vi "PC_NS_Signal disconnect_communication.vi"(8 "error in (no error)":errorcluster, 11 "PC_NS_Signal in":refnum<class "PC_NS_Signal.lvclass">) -> (0 "error out":errorcluster, 3 "PC_NS_Signal out":refnum<class "PC_NS_Signal.lvclass">)   [LabVIEW 2018, in "PC_NS_Signal.lvclass"]
uses:
  PC_NS_Signal.lvclass
  PC_NS_Signal.lvclass/PC_NS_Signal.ctl
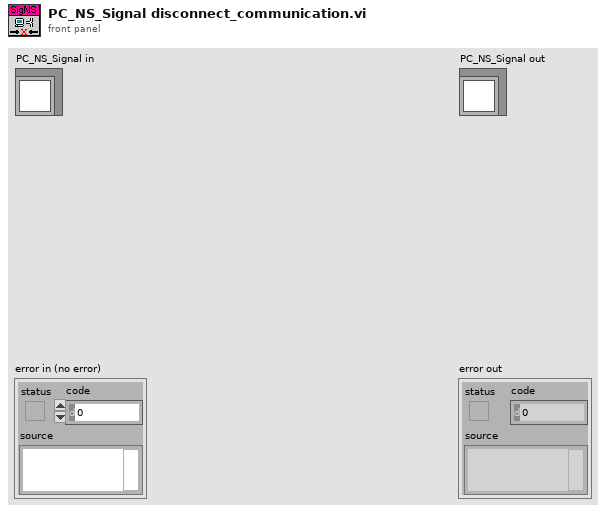
[diagram p1: front panel]
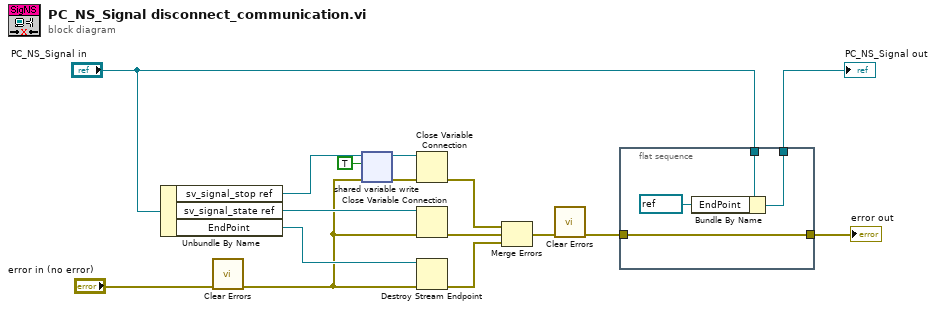
[diagram p0: block diagram]
diagram:
  n1 = Unbundle By Name("PC_NS_Signal in") -> ("sv_signal_stop ref"=w6:refnum<k21>, "sv_signal_state ref"=w16:refnum<k21>, "EndPoint"=w2:refnum<k21>)
  n2 = call <vilib>:"Clear Errors.vi"("error in (no error)"="error in (no error)") -> ("error out"=w1:errorcluster)  [unwired: 5 in, 1 out]
  n3 = shared-variable-write(w6, w1, TRUE ("data in")) -> (w4:refnum<k21>, w3:errorcluster)
  n4 = Close Variable Connection(8:w3, 11:w4) -> (0:w15:errorcluster)
  n5 = Close Variable Connection(8:w1, 11:w16) -> (0:w14:errorcluster)
  n6 = Destroy Stream Endpoint(8:w1, 11:w2) -> (0:w13:errorcluster)
  n7 = Merge Errors(w15, w14, w13) -> (w12:errorcluster)
  n8 = call <vilib>:"Clear Errors.vi"("error in (no error)"=w12) -> ("error out"=w8:errorcluster)  [unwired: 5 in, 1 out]
  n9 = flat-sequence {
    tunnel: "PC_NS_Signal in" -> [w20]
    tunnel: [w19] -> w9
    tunnel: w8 -> [w17]
    tunnel: [w17] -> w7
    frame #0 {
      n10 = Bundle By Name(cluster=w20, "EndPoint"=refnum<k21> refnum) -> (w19:refnum<class "PC_NS_Signal.lvclass">)
    }
  }
  "error out" <- w7
  "PC_NS_Signal out" <- w9
